vi "fit1.vi"() -> ()   [LabVIEW 2010]
uses:
  <vilib>/Analysis/Matrix/Datatypes/RealMatrix.ctl
  <vilib>/Analysis/baseanly.llb/Matrix Type of Inverse Matrix.ctl
  <vilib>/Analysis/7linalg.llb/Create Special Real Matrix.vi
  <vilib>/Analysis/7linalg.llb/Solve Linear Equations (single right hand).vi
  <vilib>/analysis/baseanly.llb/A x Vector.vi
  <vilib>/Analysis/polynomials.llb/1D Polynomial Evaluation (DBL).vi
  <vilib>/Analysis/NI_AALPro.lvlib
  <vilib>/Analysis/NI_AALBase.lvlib
  <vilib>/Analysis/Matrix/NI_Matrix.lvlib
panel:
  out "output matrix":T1
  out "A x Vector":dbl[](array[numeric])=[5.963812580893167e-07, -803.0325009764888] format="%#_6p"
  out "XY Graph":cluster{"Y":dbl[], "Y":dbl[]}[](graph)=[{"Y"=[5356.0, 5928.0, 6174.0, 6792.0, 7680.0, 7836.0, 7956.0], "Y"=[90.0, 125.0, 150.0, 390.0, 1900.0, 3800.0, 18000.0]}, {"Y"=[4096.0, 4137.37353515625, 4178.74755859375, 4220.12109375, 4261.4951171875, 4302.86865234375, 4344.2421875, 4385.6162109375, 4426.98974609375, 4468.36376953125, 4509.7373046875, 4551.111328125, 4592.48486328125, 4633.8583984375, 4675.232421875, 4716.60595703125, 4757.97998046875, 4799.353515625, 4840.7275390625, 4882.10107421875, 4923.474609375, 4964.8486328125, 5006.22216796875, 5047.595703125, 5088.9697265625, 5130.34326171875, 5171.71728515625, 5213.0908203125, 5254.46484375, 5295.83837890625, 5337.2119140625, 5378.5859375, 5419.95947265625, 5461.33349609375, 5502.70703125, 5544.0810546875, 5585.45458984375, 5626.828125, 5668.2021484375, 5709.57568359375, 5750.94921875, 5792.3232421875, 5833.697265625, 5875.07080078125, 5916.4443359375, 5957.818359375, 5999.19189453125, 6040.5654296875, 6081.939453125, 6123.31298828125, 6164.6865234375, 6206.060546875, 6247.4345703125, 6288.80810546875, 6330.181640625, 6371.5556640625, 6412.92919921875, 6454.302734375, 6495.6767578125, 6537.05078125, 6578.42431640625, 6619.7978515625, 6661.171875, 6702.54541015625, 6743.9189453125, 6785.29296875, 6826.6669921875, 6868.0400390625, 6909.4140625, 6950.7880859375, 6992.16162109375, 7033.53515625, 7074.9091796875, 7116.28271484375, 7157.65625, 7199.0302734375, 7240.404296875, 7281.77783203125, 7323.1513671875, 7364.525390625, 7405.89892578125, 7447.2724609375, 7488.646484375, 7530.0205078125, 7571.39404296875, 7612.767578125, 7654.1416015625, 7695.51513671875, 7736.888671875, 7778.2626953125, 7819.63671875, 7861.009765625, 7902.3837890625, 7943.7578125, 7985.13134765625, 8026.5048828125, 8067.87890625, 8109.25244140625, 8150.6259765625, 8192.0], "Y"=[4.69534807858205, 5.066941220215593, 5.4679474188668165, 5.900684614418321, 6.36767465906837, 6.871616899742052, 7.41544148295558, 8.00231191842396, 8.635620498817152, 9.319057941392794, 10.056574725995677, 10.852468861541206, 11.711340862348893, 12.638184595965276, 13.638391652337019, 14.717743537671803, 15.882530365120783, 17.139484962882502, 18.495932455184946, 19.95971352816123, 21.539339262378313, 23.243998579246778, 25.083544936967776, 27.068674284236277, 29.210934418208755, 31.52270826518445, 34.017468094286095, 36.7096343890993, 39.61489622271153, 42.75004690728647, 46.13331561695307, 49.784383336650116, 53.72435436728371, 57.976189583737835, 62.56446590890198, 67.51592233090985, 72.8591797996523, 78.62530641379942, 84.84784460251815, 91.56276256153058, 98.80910383963241, 106.62902149819548, 115.06782051293334, 124.17436857065243, 134.0016152316635, 144.60672707365276, 156.0510049238418, 168.40099095346824, 181.72852689604545, 196.11065003229874, 211.63098448539535, 228.3798143843326, 246.4541746807476, 265.9587310002393, 287.0068915930732, 309.7210967875722, 334.232641716577, 360.68404751085154, 389.22918599191524, 420.0334344517162, 453.27517518889596, 489.1476906135248, 527.8596565643768, 569.6348401804963, 614.7161411413645, 663.3658041816947, 715.8656828834245, 772.5191009401905, 833.6575540206268, 899.63460648394, 970.8323205087067, 1047.6646715803565, 1130.578605086328, 1220.0533892123574, 1316.609270537985, 1420.807929204272, 1533.253043907908, 1654.5957656762562, 1785.5416355907369, 1926.8523855487256, 2079.3448354005754, 2243.9056447366365, 2421.4920886325804, 2613.133020572427, 2819.9382014386174, 3043.110089432377, 3283.9469091238716, 3543.8407718356616, 3824.3028172082727, 4126.964535307818, 4453.579407741981, 4806.034487051747, 5186.392090678596, 5596.851830906115, 6039.790612077768, 6517.783879198568, 7033.6121912776325, 7590.257195534286, 8190.955476021941, 8839.201385340231]}, {"Y"=[4096.0, 4137.37353515625, 4178.74755859375, 4220.12109375, 4261.4951171875, 4302.86865234375, 4344.2421875, 4385.6162109375, 4426.98974609375, 4468.36376953125, 4509.7373046875, 4551.111328125, 4592.48486328125, 4633.8583984375, 4675.232421875, 4716.60595703125, 4757.97998046875, 4799.353515625, 4840.7275390625, 4882.10107421875, 4923.474609375, 4964.8486328125, 5006.22216796875, 5047.595703125, 5088.9697265625, 5130.34326171875, 5171.71728515625, 5213.0908203125, 5254.46484375, 5295.83837890625, 5337.2119140625, 5378.5859375, 5419.95947265625, 5461.33349609375, 5502.70703125, 5544.0810546875, 5585.45458984375, 5626.828125, 5668.2021484375, 5709.57568359375, 5750.94921875, 5792.3232421875, 5833.697265625, 5875.07080078125, 5916.4443359375, 5957.818359375, 5999.19189453125, 6040.5654296875, 6081.939453125, 6123.31298828125, 6164.6865234375, 6206.060546875, 6247.4345703125, 6288.80810546875, 6330.181640625, 6371.5556640625, 6412.92919921875, 6454.302734375, 6495.6767578125, 6537.05078125, 6578.42431640625, 6619.7978515625, 6661.171875, 6702.54541015625, 6743.9189453125, 6785.29296875, 6826.6669921875, 6868.0400390625, 6909.4140625, 6950.7880859375, 6992.16162109375, 7033.53515625, 7074.9091796875, 7116.28271484375, 7157.65625, 7199.0302734375, 7240.404296875, 7281.77783203125, 7323.1513671875, 7364.525390625, 7405.89892578125, 7447.2724609375, 7488.646484375, 7530.0205078125, 7571.39404296875, 7612.767578125, 7654.1416015625, 7695.51513671875, 7736.888671875, 7778.2626953125, 7819.63671875, 7861.009765625, 7902.3837890625, 7943.7578125, 7985.13134765625, 8026.5048828125, 8067.87890625, 8109.25244140625, 8150.6259765625, 8192.0], "Y"=[70.13241598902006, 70.14991508063308, 70.16972696793826, 70.19215679520558, 70.21755109680261, 70.24630099778989, 70.27885026738034, 70.31570146373117, 70.35742217191057, 70.40465696483712, 70.45813335656239, 70.51867754192808, 70.5872220273107, 70.66482483139148, 70.75268413534941, 70.85215315519824, 70.96476865863028, 71.09226515861997, 71.23661243935105, 71.40003374916516, 71.58505157835067, 71.79452258760863, 72.03167306614652, 72.30016355113466, 72.60413951450101, 72.94828281830102, 73.33791037740544, 73.77902326658517, 74.27843655286104, 74.84384223953847, 75.48396764838017, 76.20869626524919, 77.02919041816058, 77.95812650533226, 79.00981207453964, 80.2004953647592, 81.54851537508401, 83.07467947383356, 84.80255151441277, 86.75874431993374, 88.97345271235513, 91.48087161471065, 94.31965611758208, 97.53355719967843, 101.17218304414644, 105.29171374725794, 109.95559864978115, 115.23582716598546, 121.21392560801647, 127.98196912533454, 135.6444258810149, 144.31960360347287, 154.14124132624593, 165.26070885653922, 177.8496407803733, 192.10240921449576, 208.23853643618506, 226.50709170241154, 247.1901400667071, 270.60653734820835, 297.1171740258749, 327.13125513932926, 361.11219573549795, 399.5833729742813, 443.13860886749023, 492.45039282464865, 548.2789294824112, 611.4838478197498, 683.0431394219241, 764.0592822953265, 855.7808867301568, 959.623721922506, 1077.1911130636981, 1210.2938424979777, 1360.986417943671, 1531.595520889305, 1724.7513103092003, 1943.4306781871967, 2191.0090507903105, 2471.309018679425, 2788.647784337467, 3147.923631564772, 3554.683751127339, 4015.198873955689, 4536.566399416905, 5126.833898058182, 5795.115053538469, 6551.702785566102, 7408.275407137733, 8378.058332022358, 9476.002012563955, 10719.01221526792, 12126.322467375601, 13719.614489966027, 15523.443893120488, 17565.65369288437, 19877.775447615877, 22495.420641167384, 25458.993946507337, 28814.252701905494]}]
  in  "Code":dbl[](array[numeric])=[7956.0, 7836.0, 7680.0, 6792.0, 6174.0, 5928.0, 5356.0] caption="Код"
  in  "mV":dbl[](array[numeric])=[18000.0, 3800.0, 1900.0, 390.0, 150.0, 125.0, 90.0] caption="ЧР"
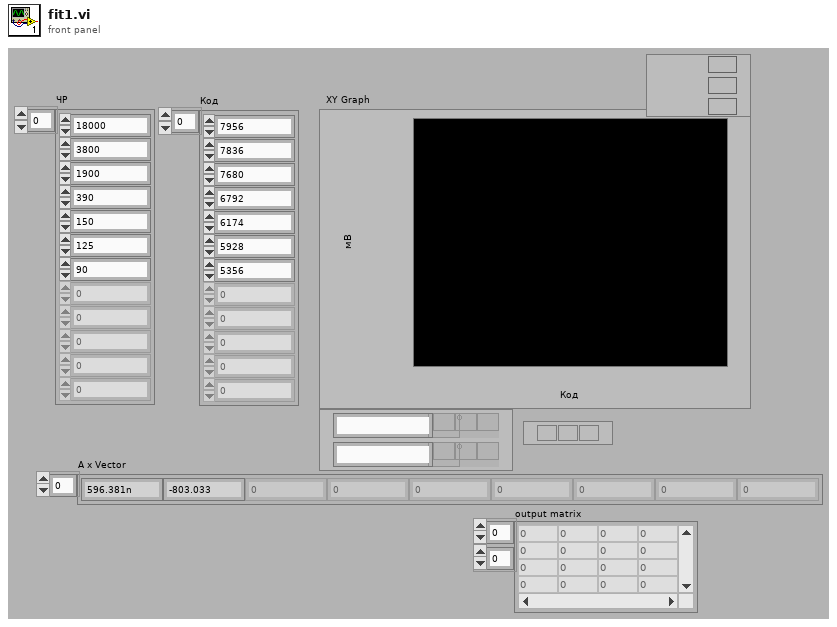
[diagram p1: front panel]
types:
  T1 = typedef "NI_Matrix.lvlib/RealMatrix.ctl" = dbl[][]
  T2 = enum32{"Identity", "Diagonal", "Toepliz", "Vandermonde", "Companion"}
  T3 = typedef "NI_AALBase.lvlib/Matrix Type of Inverse Matrix.ctl" = enum32{"General", "Positive Definite", "Lower Triangular", "Upper Triangular"}
  T4 = enum32{"General", "Positive Definite", "Lower Triangular", "Upper Triangular"}
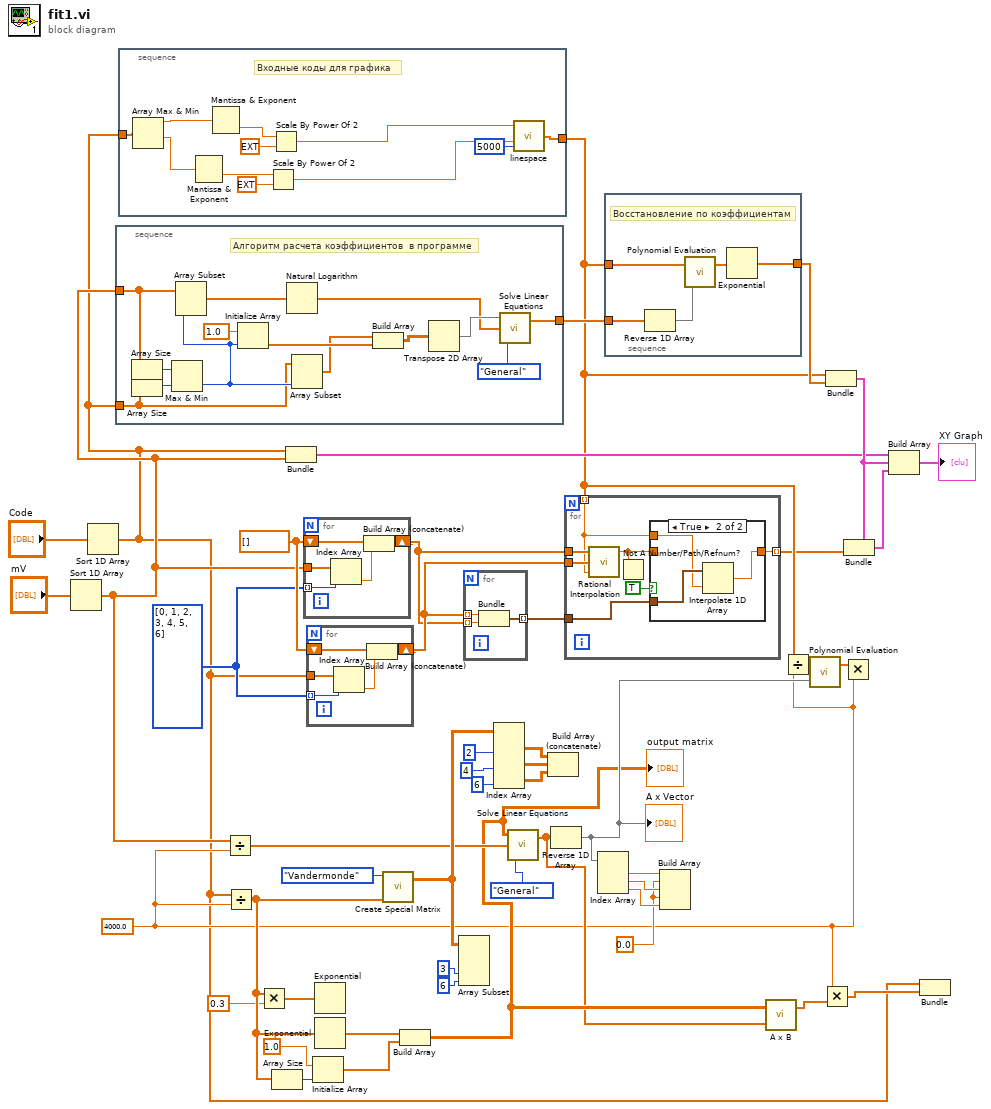
[diagram p0: block diagram]
diagram:
  w25 = 0.0 ("element")
  w8 = 4000.0 ("element")
  w42 = dbl[] []
  w41 = i32[] [0, 1, 2, 3, 4, 5, 6]
  n1 = Sort 1D Array(array="mV") -> (sorted array=w37:dbl[])
  n2 = Sort 1D Array(array="Code") -> (sorted array=w6:dbl[])
  n3 = stacked-sequence {
    tunnel: [w53] -> w47
    tunnel: w37 -> [w52]
    tunnel: w6 -> [w51]
    frame #0 {
      # "Алгоритм расчета коэффициентов  в программе"
      n4 = Array Size(array=w52) -> (size(s)=w61:i32)
      n5 = Array Size(array=w51) -> (size(s)=w60:i32)
      n6 = Max & Min(x=w61, y=w60) -> (min(x,y)=w58:i32)  [unwired: 1 out]
      n7 = Array Subset(array=w52, length=w58) -> (w59:dbl[])  [unwired: 1 in]
      n8 = Initialize Array(1.0, w58) -> (w54:dbl[])
      n9 = Natural Logarithm(1:w59) -> (0:w55:dbl[])
      n10 = Array Subset(array=w51, length=w58) -> (w49:dbl[])  [unwired: 1 in]
      n11 = Build Array(w49, w54) -> (w50:dbl[][])
      n12 = Transpose 2D Array(2D array=w50) -> (transposed array=w56:dbl[][])
      n13 = call-poly <vilib>:"Solve Linear Equations.vi"("matrix type"=T4."General", "Known Vector"=w55, "Input Matrix"=w56) -> ("Solution Vector"=w53:dbl[])  [unwired: 1 out]
    }
  }
  n14 = stacked-sequence {
    tunnel: w6 -> [w73]
    tunnel: [w72] -> w36
    frame #0 {
      # "Входные коды для графика"
      n15 = Array Max & Min(array=w73) -> (max value=w70:dbl, min value=w66:dbl)  [unwired: 2 out]
      n16 = Mantissa & Exponent(0:w66) -> (2:w67:dbl)  [unwired: 1 out]
      n17 = Mantissa & Exponent(0:w70) -> (2:w69:dbl)  [unwired: 1 out]
      n18 = Scale By Power Of 2(n=w67, x=ext 1.0) -> (x*2^n=w63:ext)
      n19 = Scale By Power Of 2(n=w69, x=ext 2.0) -> (x*2^n=w64:ext)
      n20 = call "linespace.vi"("N"=5000, "a"=w63, "b"=w64) -> ("Array"=w72:sgl[])
    }
  }
  n21 = Divide(x=w37, y=w8) -> (x/y=w19:dbl[])
  n22 = Divide(x=w6, y=w8) -> (x/y=w17:dbl[])
  n23 = Multiply(x=w17, y=0.3 ("element")) -> (x*y=w15:dbl[])
  n24 = Array Size(array=w17) -> (size(s)=w18:i32)
  n25 = Bundle(w6, w37) -> (w40:cluster{dbl[], dbl[]})  [unwired: 1 in]
  n26 = for {
    tunnel: w41 -> [w78] mode=indexing
    shift-right: [w76] -> w2
    shift-left: w42 -> [w75]
    tunnel: w37 -> [w74]
    n27 = Index Array(array=w74, index=w78) -> (element=w77:dbl)
    n28 = Build Array (concatenate)(w75, w77) -> (w76:dbl[])
  }
  n29 = for {
    tunnel: w41 -> [w83] mode=indexing
    shift-right: [w81] -> w3
    shift-left: w42 -> [w80]
    tunnel: w6 -> [w79]
    n30 = Index Array(array=w79, index=w83) -> (element=w82:dbl)
    n31 = Build Array (concatenate)(w80, w82) -> (w81:dbl[])
  }
  n32 = Initialize Array(1.0 ("element"), w18) -> (w12:dbl[])
  n33 = Exponential(1:w15) -> ()  [unwired: 1 out]
  n34 = Exponential(1:w17) -> (0:w13:dbl[])
  n35 = call-poly <vilib>:"Create Special Matrix.vi"("matrix type"=T2."Vandermonde", "Input Vector1"=w17) -> ("Special Matrix"=w22:T1)  [unwired: 3 in, 1 out]
  n36 = Build Array(w13, w12) -> (w11:T1)
  "output matrix" <- w11
  n37 = Array Subset(array=w22, index (col)=3 ("column 1"), length (col)=6 ("column N")) -> ()  [unwired: 2 in, 1 out]
  n38 = for {
    tunnel: w3 -> [w84] mode=indexing
    tunnel: w2 -> [w85] mode=indexing
    tunnel: [w86] -> w1 mode=indexing
    n39 = Bundle("Numeric"=w84, "Numeric"=w85) -> (w86:cluster{"Numeric":dbl, "Numeric":dbl})  [unwired: 1 in]
  }
  n40 = Index Array(array=w22, index (col) #1=2 ("index (col)"), index (col) #2=4 ("index (col)"), index (col) #3=6 ("index (col)")) -> (element #1=w33:T1, element #2=w32:T1, element #3=w31:T1)  [unwired: 3 in]
  n41 = call-poly <vilib>:"Solve Linear Equations.vi"("matrix type"=Matrix_Type_of_Inverse_Matrix."General", "Known Vector"=w19, "Input Matrix"=w11) -> ("Solution Vector"=w10:dbl[])  [unwired: 1 out]
  n42 = Build Array (concatenate)(w33, w32, w31) -> ()  [unwired: 1 out]
  n43 = Reverse 1D Array(array=w10) -> (reversed array=w23:dbl[])
  "A x Vector" <- w23
  n44 = for {
    tunnel: w2 -> [w91]
    tunnel: w3 -> [w90]
    tunnel: w36 -> [w88] mode=indexing
    tunnel: [w93] -> w5 mode=indexing
    tunnel: w1 -> [w89]
    n45 = call <vilib>:"Rational Interpolation.vi"("x value"=w88, "X"=w90, "Y"=w91) -> ("interpolation value"=w92:dbl)  [unwired: 2 out]
    n46 = Not A Number/Path/Refnum?(number/path/refnum=w92) -> ()  [unwired: 1 out]
    n47 = case shown="True" TRUE {
      tunnel: [w94 w95] -> w93
      tunnel: w92 -> [w94 _]
      tunnel: w89 -> [_ w97]
      tunnel: w88 -> [_ w96]
      frame False {
      }
      frame True {
        n48 = Interpolate 1D Array(1:w96, 2:w97) -> (0:w95:dbl)
      }
    }
  }
  n49 = Index Array(array=w23) -> (element #1=w28:dbl, element #2=w27:dbl, element #3=w26:dbl)  [unwired: 3 in]
  n50 = stacked-sequence {
    tunnel: w47 -> [w99]
    tunnel: w36 -> [w102]
    tunnel: [w101] -> w46
    frame #0 {
      # "Восстановление по коэффициентам"
      n51 = Reverse 1D Array(array=w99) -> (reversed array=w100:dbl[])
      n52 = call-poly <vilib>:"Polynomial Evaluation.vi"("P(x)"=w100, "A"=w102) -> ("P(A)"=w98:dbl[])  [unwired: 1 out]
      n53 = Exponential(1:w98) -> (0:w101:dbl[])
    }
  }
  n54 = Build Array(w28, w25, w27, w25, w26) -> ()  [unwired: 1 out]
  n55 = call-poly <vilib>:"A x B.vi"("Vector"=w10, "A"=w11) -> ("A x Vector"=w9:dbl[])  [unwired: 1 out]
  n56 = Divide(x=w36, y=w8) -> (x/y=w35:dbl[])
  n57 = call-poly <vilib>:"Polynomial Evaluation.vi"("P(x)"=w23, "A"=w35) -> ("P(A)"=w24:dbl[])  [unwired: 1 out]
  n58 = Multiply(x=w8, y=w9) -> (x*y=w7:dbl[])
  n59 = Bundle("Array"=w36, w46) -> (w45:cluster{"Array":sgl[], dbl[]})  [unwired: 1 in]
  n60 = Multiply(x=w24, y=w8) -> ()  [unwired: 1 out]
  n61 = Bundle(cluster=w45, w5) -> (w4:cluster{"Array":sgl[], dbl[]})  [unwired: 1 in]
  n62 = Build Array(w40, w45, w4) -> (→"XY Graph":cluster{"Array":dbl[], dbl[]}[])
  n63 = Bundle(w6, w7) -> ()  [unwired: 1 in, 1 out]
